vi "move to cache.vi"(7 "Time Stamp":timestamp, 8 "sample counter":i32, 9 "output type order":T2[](array[typedef]), 10 "data table in":T1, 11 "cache in":T3) -> (2 "data table out":T1, 3 "cache out":T3)   [LabVIEW 2013, in "TDMS datalogger runtime.lvclass"]
uses:
  TDMS datalogger runtime.lvclass
  data cache.ctl
  <vilib>/NI/Tag Bus/tag/Data Type.ctl
  <vilib>/NI/Tag Bus/table/data table.ctl
  <vilib>/NI/Tag Bus/tag/tag descriptor.lvclass
  <vilib>/NI/Tag Bus/table/data table.lvlib
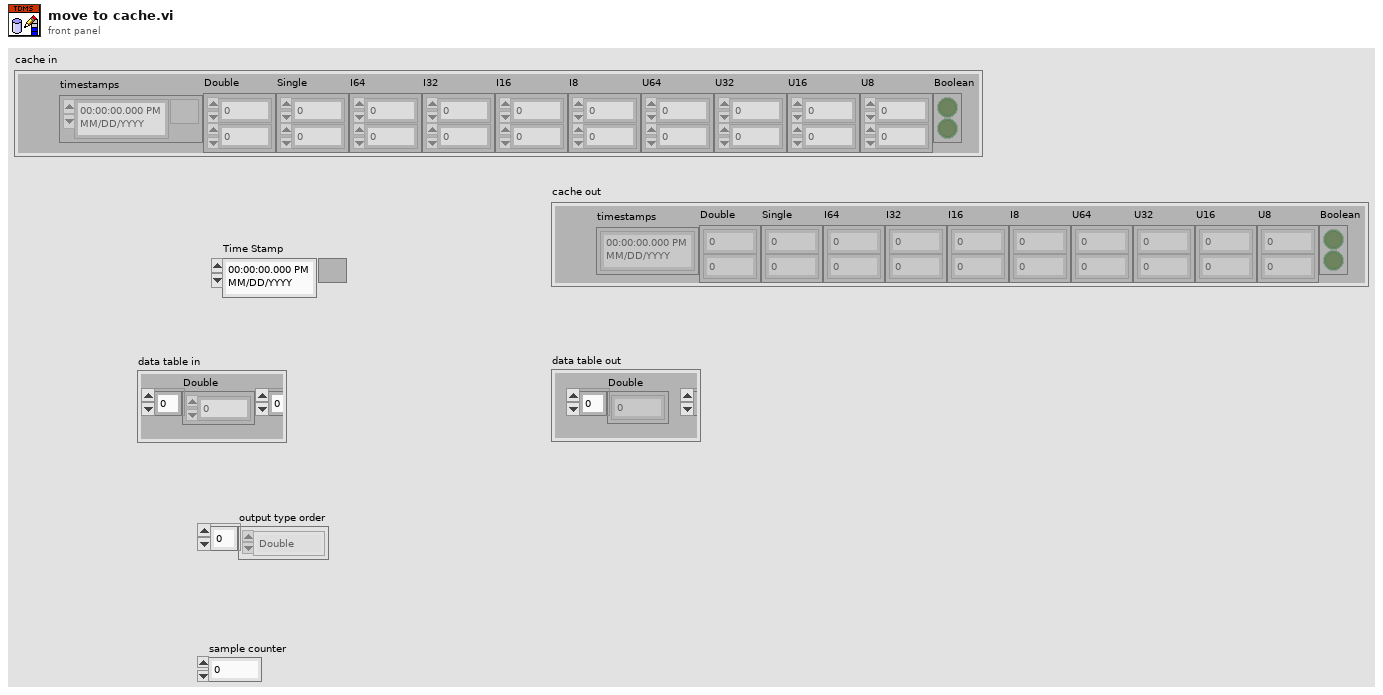
[diagram p1: front panel]
types:
  T1 = typedef "tag bus.lvlib/data table.lvlib/data table.ctl" = cluster{"Double":dbl[], "Single":sgl[], "I64":i64[], "I32":i32[], "I16":i16[], "I8":i8[], "U64":u64[], "U32":u32[], "U16":u16[], "U8":u8[], "Boolean":bool[], "String":string[], "Array of Double":cluster{"DBL Array":dbl[]}[], "Array of Single":cluster{"SGL Array":sgl[]}[], "Array of I64":cluster{"I64 Array":i64[]}[], "Array of I32":cluster{"I32 Array":i32[]}[], "Array of I16":cluster{"I16 Array":i16[]}[], "Array of I8":cluster{"I8 Array":i8[]}[], "Array of U64":cluster{"U64 Array":u64[]}[], "Array of U32":cluster{"U32 Array":u32[]}[], "Array of U16":cluster{"U16 Array":u16[]}[], "Array of U8":cluster{"U8 Array":u8[]}[], "Array of Boolean":cluster{"Boolean Array":bool[]}[], "Array of String":cluster{"String Array":string[]}[]}
  T2 = typedef "tag bus.lvlib/tag descriptor.lvclass/Data Type.ctl" = enum16{"Double", "Single", "I64", "I32", "I16", "I8", "U64", "U32", "U16", "U8", "Boolean", "String", "Array of Double", "Array of Single", "Array of I64", "Array of I32", "Array of I16", "Array of I8", "Array of U64", "Array of U32", "Array of U16", "Array of U8", "Array of Boolean", "Array of String"}
  T3 = typedef "TDMS datalogger runtime.lvclass/data cache.ctl" = cluster{"timestamps":timestamp[], "Double":dbl[][], "Single":sgl[][], "I64":i64[][], "I32":i32[][], "I16":i16[][], "I8":i8[][], "U64":u64[][], "U32":u32[][], "U16":u16[][], "U8":u8[][], "Boolean":bool[][]}
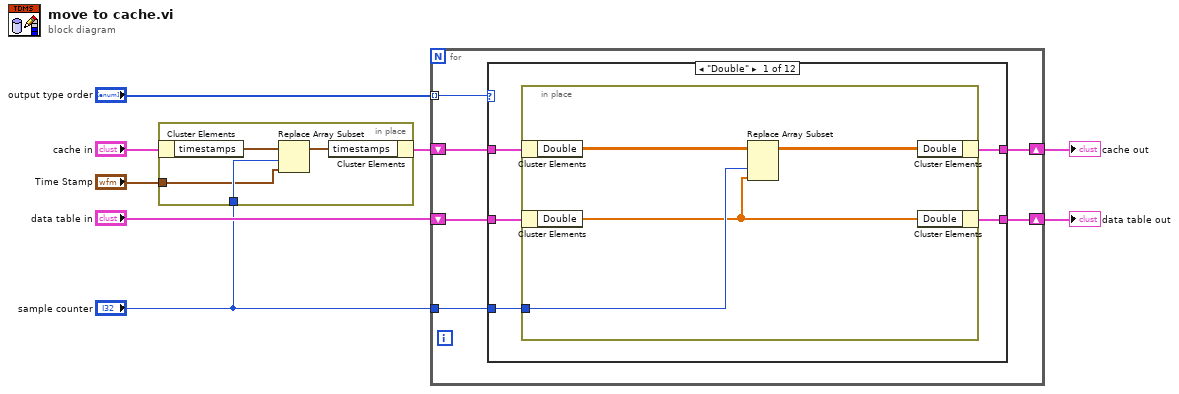
[diagram p0: block diagram]
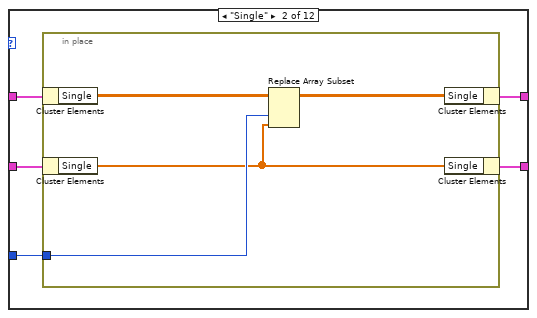
[diagram p2: hidden frame]
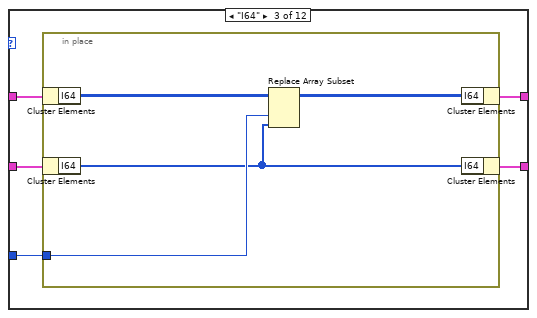
[diagram p3: hidden frame]
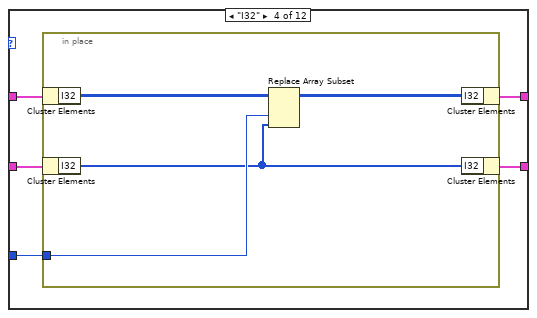
[diagram p4: hidden frame]
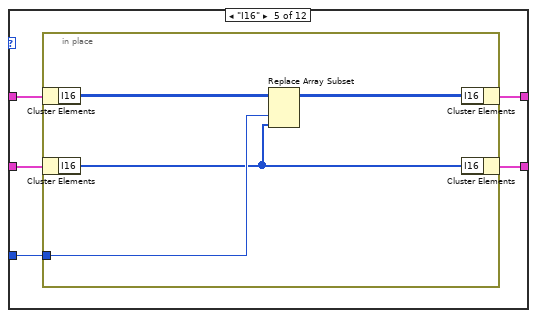
[diagram p5: hidden frame]
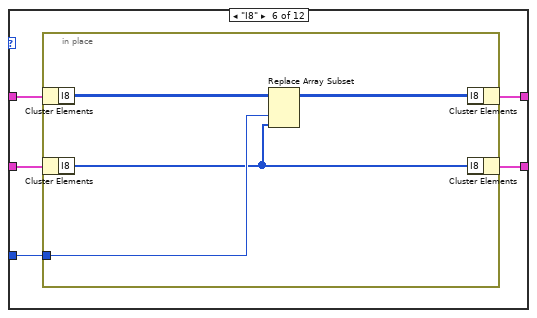
[diagram p6: hidden frame]
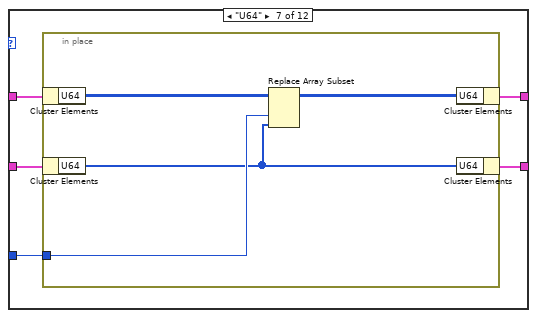
[diagram p7: hidden frame]
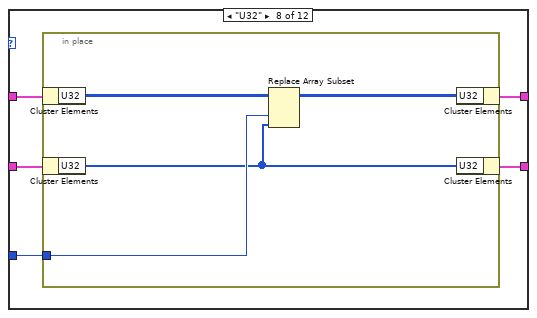
[diagram p8: hidden frame]
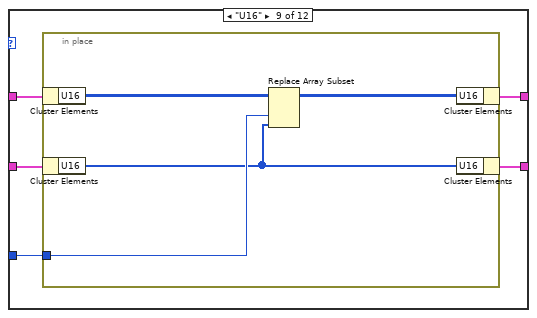
[diagram p9: hidden frame]
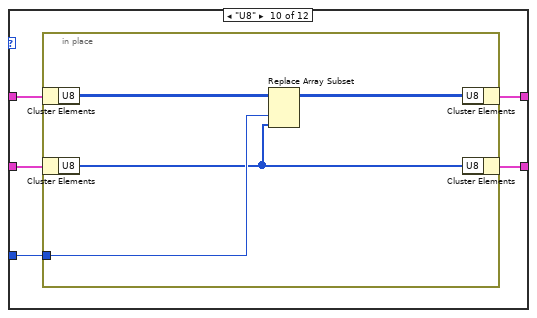
[diagram p10: hidden frame]
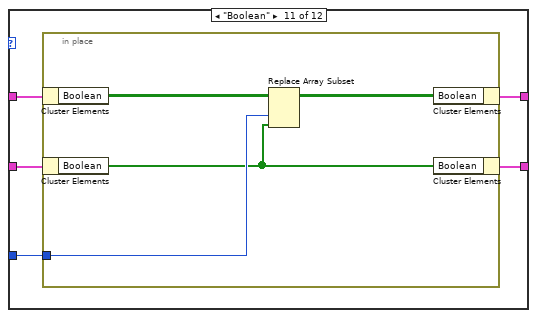
[diagram p11: hidden frame]
diagram:
  n1 = in-place {
    in-place-border: "sample counter" -> [w10]
    in-place-border: "Time Stamp" -> [w9]
    n2 = in-place-cluster #1("cache in") -> ("timestamps"=w12:timestamp[])
    n3 = Replace Array Subset(array=w12, new element=w9, index=w10) -> (w11:timestamp[])
    n4 = in-place-cluster #1("timestamps"=w11) -> (w3:T3)
  }
  n5 = for {
    shift-right: [w17] -> w8
    shift-left: w3 -> [w16]
    tunnel: "output type order" -> [w18] mode=indexing
    tunnel: "sample counter" -> [w13]
    shift-right: [w14] -> w5
    shift-left: "data table in" -> [w15]
    n6 = case shown="\"Double\"" w18 {
      tunnel: [w22 w31 w40 w49 w58 w67 w76 w85 w94 w103 w112 w119] -> w17
      tunnel: w16 -> [w23 w32 w41 w50 w59 w68 w77 w86 w95 w104 w113 w119]
      tunnel: w15 -> [w21 w30 w39 w48 w57 w66 w75 w84 w93 w102 w111 w118]
      tunnel: [w20 w29 w38 w47 w56 w65 w74 w83 w92 w101 w110 w118] -> w14
      tunnel: w13 -> [w19 w28 w37 w46 w55 w64 w73 w82 w91 w100 w109 _]
      frame "Double" {
        n7 = in-place {
          in-place-border: w19 -> [w25]
          n8 = in-place-cluster #2(w23) -> ("Double"=w27:dbl[][])
          n9 = in-place-cluster #3(w21) -> ("Double"=w24:dbl[])
          n10 = Replace Array Subset(array=w27, new element=w24, index (col)=w25) -> (w26:dbl[][])  [unwired: 1 in]
          n11 = in-place-cluster #2("Double"=w26) -> (w22:T3)
          n12 = in-place-cluster #3("Double"=w24) -> (w20:T1)
        }
      }
      frame "Single" {
        n13 = in-place {
          in-place-border: w28 -> [w34]
          n14 = in-place-cluster #4(w32) -> ("Single"=w36:sgl[][])
          n15 = in-place-cluster #5(w30) -> ("Single"=w33:sgl[])
          n16 = Replace Array Subset(array=w36, new element=w33, index (col)=w34) -> (w35:sgl[][])  [unwired: 1 in]
          n17 = in-place-cluster #4("Single"=w35) -> (w31:T3)
          n18 = in-place-cluster #5("Single"=w33) -> (w29:T1)
        }
      }
      frame "I64" {
        n19 = in-place {
          in-place-border: w37 -> [w43]
          n20 = in-place-cluster #6(w41) -> ("I64"=w45:i64[][])
          n21 = in-place-cluster #7(w39) -> ("I64"=w42:i64[])
          n22 = Replace Array Subset(array=w45, new element=w42, index (col)=w43) -> (w44:i64[][])  [unwired: 1 in]
          n23 = in-place-cluster #6("I64"=w44) -> (w40:T3)
          n24 = in-place-cluster #7("I64"=w42) -> (w38:T1)
        }
      }
      frame "I32" {
        n25 = in-place {
          in-place-border: w46 -> [w52]
          n26 = in-place-cluster #8(w50) -> ("I32"=w54:i32[][])
          n27 = in-place-cluster #9(w48) -> ("I32"=w51:i32[])
          n28 = Replace Array Subset(array=w54, new element=w51, index (col)=w52) -> (w53:i32[][])  [unwired: 1 in]
          n29 = in-place-cluster #8("I32"=w53) -> (w49:T3)
          n30 = in-place-cluster #9("I32"=w51) -> (w47:T1)
        }
      }
      frame "I16" {
        n31 = in-place {
          in-place-border: w55 -> [w61]
          n32 = in-place-cluster #10(w59) -> ("I16"=w63:i16[][])
          n33 = in-place-cluster #11(w57) -> ("I16"=w60:i16[])
          n34 = Replace Array Subset(array=w63, new element=w60, index (col)=w61) -> (w62:i16[][])  [unwired: 1 in]
          n35 = in-place-cluster #10("I16"=w62) -> (w58:T3)
          n36 = in-place-cluster #11("I16"=w60) -> (w56:T1)
        }
      }
      frame "I8" {
        n37 = in-place {
          in-place-border: w64 -> [w70]
          n38 = in-place-cluster #12(w68) -> ("I8"=w72:i8[][])
          n39 = in-place-cluster #13(w66) -> ("I8"=w69:i8[])
          n40 = Replace Array Subset(array=w72, new element=w69, index (col)=w70) -> (w71:i8[][])  [unwired: 1 in]
          n41 = in-place-cluster #12("I8"=w71) -> (w67:T3)
          n42 = in-place-cluster #13("I8"=w69) -> (w65:T1)
        }
      }
      frame "U64" {
        n43 = in-place {
          in-place-border: w73 -> [w79]
          n44 = in-place-cluster #14(w77) -> ("U64"=w81:u64[][])
          n45 = in-place-cluster #15(w75) -> ("U64"=w78:u64[])
          n46 = Replace Array Subset(array=w81, new element=w78, index (col)=w79) -> (w80:u64[][])  [unwired: 1 in]
          n47 = in-place-cluster #14("U64"=w80) -> (w76:T3)
          n48 = in-place-cluster #15("U64"=w78) -> (w74:T1)
        }
      }
      frame "U32" {
        n49 = in-place {
          in-place-border: w82 -> [w88]
          n50 = in-place-cluster #16(w86) -> ("U32"=w90:u32[][])
          n51 = in-place-cluster #17(w84) -> ("U32"=w87:u32[])
          n52 = Replace Array Subset(array=w90, new element=w87, index (col)=w88) -> (w89:u32[][])  [unwired: 1 in]
          n53 = in-place-cluster #16("U32"=w89) -> (w85:T3)
          n54 = in-place-cluster #17("U32"=w87) -> (w83:T1)
        }
      }
      frame "U16" {
        n55 = in-place {
          in-place-border: w91 -> [w97]
          n56 = in-place-cluster #18(w95) -> ("U16"=w99:u16[][])
          n57 = in-place-cluster #19(w93) -> ("U16"=w96:u16[])
          n58 = Replace Array Subset(array=w99, new element=w96, index (col)=w97) -> (w98:u16[][])  [unwired: 1 in]
          n59 = in-place-cluster #18("U16"=w98) -> (w94:T3)
          n60 = in-place-cluster #19("U16"=w96) -> (w92:T1)
        }
      }
      frame "U8" {
        n61 = in-place {
          in-place-border: w100 -> [w106]
          n62 = in-place-cluster #20(w104) -> ("U8"=w108:u8[][])
          n63 = in-place-cluster #21(w102) -> ("U8"=w105:u8[])
          n64 = Replace Array Subset(array=w108, new element=w105, index (col)=w106) -> (w107:u8[][])  [unwired: 1 in]
          n65 = in-place-cluster #20("U8"=w107) -> (w103:T3)
          n66 = in-place-cluster #21("U8"=w105) -> (w101:T1)
        }
      }
      frame "Boolean" {
        n67 = in-place {
          in-place-border: w109 -> [w115]
          n68 = in-place-cluster #22(w113) -> ("Boolean"=w117:bool[][])
          n69 = in-place-cluster #23(w111) -> ("Boolean"=w114:bool[])
          n70 = Replace Array Subset(array=w117, new element=w114, index (col)=w115) -> (w116:bool[][])  [unwired: 1 in]
          n71 = in-place-cluster #22("Boolean"=w116) -> (w112:T3)
          n72 = in-place-cluster #23("Boolean"=w114) -> (w110:T1)
        }
      }
      frame Default {
      }
    }
  }
  "cache out" <- w8
  "data table out" <- w5
